vi "BasicExampleExportCSV.vi"() -> ()   [LabVIEW 2025]
uses:
  PalmSens/PalmSens.lvclass
  E:/PSCode/PalmSens_SDK/labview/PalmSens/Libraries/PalmSens.Core.Simplified.LabVIEW.dll
  PalmSens/Libraries/PalmSens.Core.Simplified.LabVIEW.dll
  <vilib>/Utility/file.llb/Write Delimited Spreadsheet (DBL).vi
panel:
  out "LSV Method Indicator":refnum<k24>
  out "Array":string[](array[string])
  out "Is Measuring":bool
  in  "PalmSens.lvclass":refnum<class "PalmSens.lvclass">
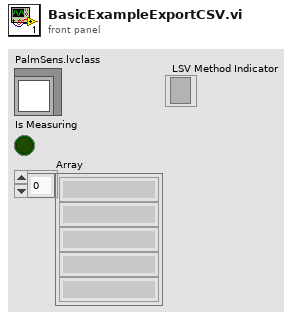
[diagram p1: front panel]
types:
  T1 = enum16{"open", "replace", "create", "open or create", "replace or create", "replace or create with confirmation"}
  T2 = typedef "MeasurementResults.ctl" = T3[]
  T3 = typedef "LiveCurveResult.ctl" = cluster{"X Label":string, "Y Label":string, "Name":string, "Index":i16, "Curve Values":cluster{"Values":cluster{"X Value":dbl, "Y Value":dbl}[], "Index":i16}}
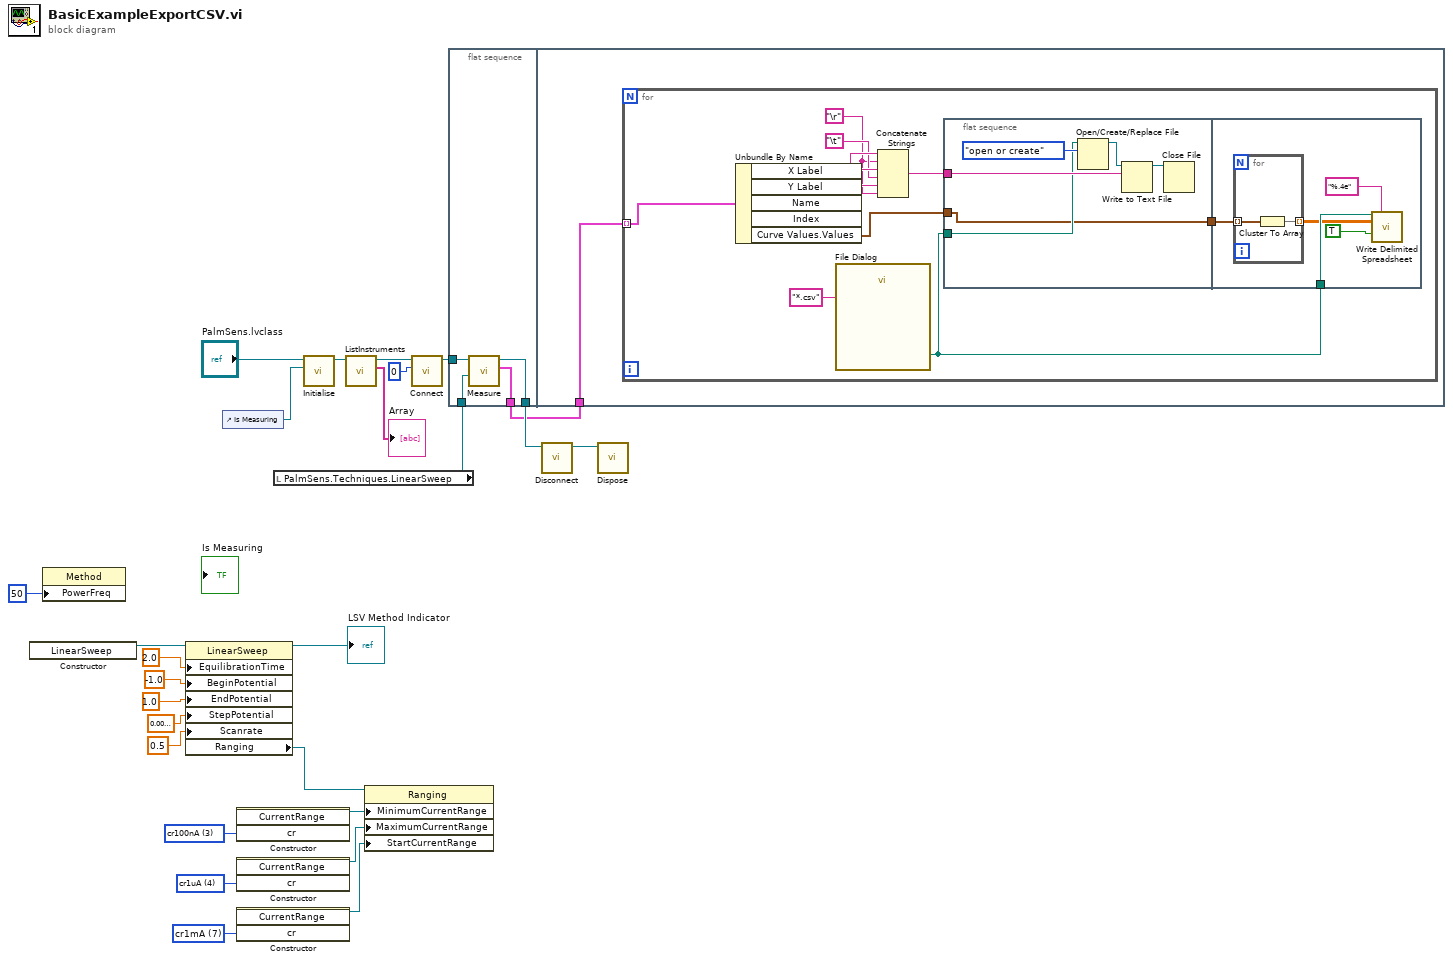
[diagram p0: block diagram]
diagram:
  w17 = 4 items=["cr100pA"=0, "cr1nA"=1, "cr10nA"=2, "cr100nA"=3, "cr1uA"=4, "cr10uA"=5, "cr100uA"=6, "cr1mA"=7, "cr10mA"=8, "cr100mA"=9, "cr2uA"=10, "cr4uA"=11, "cr8uA"=12, "cr16uA"=13, "cr32uA"=14, "cr125uA"=17, "cr250uA"=18, "cr500uA"=19, "cr5mA"=20, "cr6uA"=21, "cr13uA"=22, "cr25uA"=23, "cr50uA"=24, "cr200uA"=25, "cr63uA"=26] ("cr")
  w18 = 7 items=["cr100pA"=0, "cr1nA"=1, "cr10nA"=2, "cr100nA"=3, "cr1uA"=4, "cr10uA"=5, "cr100uA"=6, "cr1mA"=7, "cr10mA"=8, "cr100mA"=9, "cr2uA"=10, "cr4uA"=11, "cr8uA"=12, "cr16uA"=13, "cr32uA"=14, "cr125uA"=17, "cr250uA"=18, "cr500uA"=19, "cr5mA"=20, "cr6uA"=21, "cr13uA"=22, "cr25uA"=23, "cr50uA"=24, "cr200uA"=25, "cr63uA"=26] ("cr")
  w20 = 3 items=["cr100pA"=0, "cr1nA"=1, "cr10nA"=2, "cr100nA"=3, "cr1uA"=4, "cr10uA"=5, "cr100uA"=6, "cr1mA"=7, "cr10mA"=8, "cr100mA"=9, "cr2uA"=10, "cr4uA"=11, "cr8uA"=12, "cr16uA"=13, "cr32uA"=14, "cr125uA"=17, "cr250uA"=18, "cr500uA"=19, "cr5mA"=20, "cr6uA"=21, "cr13uA"=22, "cr25uA"=23, "cr50uA"=24, "cr200uA"=25, "cr63uA"=26] ("cr")
  n1 = constructor class="LinearSweep"() -> (reference out=w16:refnum<k24>)  [unwired: 3 in, 2 out]
  n2 = property class="Method"("PowerFreq"=50) -> ()  [unwired: 2 in, 2 out]
  n3 = property class="LinearSweep"(reference=w16, "EquilibrationTime"=sgl 2.0, "BeginPotential"=sgl -1.0, "EndPotential"=sgl 1.0, "StepPotential"=sgl 0.01, "Scanrate"=sgl 0.5) -> (reference out=→"LSV Method Indicator":refnum<k24>, "Ranging"=w5:refnum<k24>)  [unwired: 1 in, 1 out]
  n4 = control-ref of="Is Measuring"() -> (w25:refnum<vi>)
  n5 = constructor class="CurrentRange"("cr"=w20) -> (reference out=w19:refnum<k24>)  [unwired: 3 in, 3 out]
  n6 = constructor class="CurrentRange"("cr"=w17) -> (reference out=w7:refnum<k24>)  [unwired: 3 in, 3 out]
  n7 = constructor class="CurrentRange"("cr"=w18) -> (reference out=w6:refnum<k24>)  [unwired: 3 in, 3 out]
  n8 = local read "LSV Method Indicator"() -> (w11:refnum<k24>)
  n9 = call-dynamic "Initialise.vi"("Is Measuring Refnum"=w25, "PalmSens in"="PalmSens.lvclass") -> ("PalmSens out"=w24:refnum<class "PalmSens.lvclass">)  [unwired: 8 in, 1 out]
  n10 = call-dynamic "ListInstruments.vi"("PalmSens in"=w24) -> ("Array"=→"Array":string[], "PalmSens out"=w22:refnum<class "PalmSens.lvclass">)  [unwired: 8 in, 1 out]
  n11 = property class="Ranging"(reference=w5, "MinimumCurrentRange"=w19, "MaximumCurrentRange"=w7, "StartCurrentRange"=w6) -> ()  [unwired: 1 in, 2 out]
  n12 = call-dynamic "Connect.vi"("Instrument Index"=0, "PalmSens in"=w22) -> ("PalmSens out"=w10:refnum<class "PalmSens.lvclass">)  [unwired: 8 in, 1 out]
  n13 = flat-sequence {
    tunnel: w11 -> [w27]
    tunnel: w10 -> [w30]
    tunnel: [w28] -> w8
    tunnel: [w29] -> w9
    tunnel: w8 -> [w31]
    frame #0 {
      n14 = call-dynamic "Measure.vi"("Method .NET Refnum"=w27, "PalmSens in"=w30) -> ("Curves"=w28:T2, "PalmSens out"=w29:refnum<class "PalmSens.lvclass">)  [unwired: 2 in, 2 out]
    }
    frame #1 {
      n15 = for {
        tunnel: w31 -> [w33] mode=indexing
        w34 = "\r"
        n16 = Unbundle By Name(w33) -> ("X Label"=w41:string, "Y Label"=w39:string, "Name"=w42:string, "Curve Values.Values"=w32:cluster{"X Value":dbl, "Y Value":dbl}[])  [unwired: 1 out]
        n17 = call "File Dialog"("pattern (all files)"="*.csv") -> ("selected path"=w36:path)  [unwired: 11 in, 3 out]
        n18 = Concatenate Strings(w42, w34, w41, "\t", w39, w34) -> (w37:string)
        n19 = flat-sequence {
          tunnel: [w43] -> w38
          tunnel: w37 -> [w46]
          tunnel: w36 -> [w44]
          tunnel: w32 -> [w43]
          tunnel: w36 -> [w53]
          tunnel: w38 -> [w52]
          frame #0 {
            n20 = Open/Create/Replace File(file path (use dialog)=w44, operation (0:open)=T1."open or create") -> (refnum out=w47:refnum<file>)  [unwired: 4 in, 2 out]
            n21 = Write to Text File(file (use dialog)=w47, text=w46) -> (refnum out=w48:refnum<file>)  [unwired: 2 in, 2 out]
            n22 = Close File(refnum=w48) -> ()  [unwired: 1 in, 2 out]
          }
          frame #1 {
            n23 = for {
              tunnel: w52 -> [w55] mode=indexing
              tunnel: [w54] -> w51 mode=indexing
              n24 = Cluster To Array(cluster=w55) -> (array=w54:dbl[])
            }
            n25 = call-poly <vilib>:"Write Delimited Spreadsheet.vi"("file path (dialog if empty)"=w53, "format (%.3f)"="%.4e", "2D data"=w51, "append to file? (new file:F)"=TRUE) -> ()  [unwired: 10 in, 2 out]
          }
        }
      }
    }
  }
  n26 = call-dynamic "Disconnect.vi"("PalmSens in"=w9) -> ("PalmSens out"=w12:refnum<class "PalmSens.lvclass">)  [unwired: 9 in, 1 out]
  n27 = call-dynamic "Dispose.vi"("PalmSens in"=w12) -> ()  [unwired: 9 in, 2 out]
